vi "To and From CSV.vi"() -> (0 "error out":errorcluster, 1 "Pass":bool, 2 "Lines Equal":bool, 3 "Class Equal":bool)   [LabVIEW 2017, in "J1939 tests.lvlib"]
uses:
  J1939 tests.lvlib
  <vilib>/NI/DCAF/Engines/Standard Engine/Execution Engine/Configuration/Standard Engine Configuration.lvclass
  C:/Program Files (x86)/National Instruments/LabVIEW 2017/vi.lib/NI/Module Execution Interface/Engine Configuration/engine configuration.lvclass
  editor node/J1939 editor node.lvclass
  module/configuration/J1939 configuration.lvclass
  C:/Program Files (x86)/National Instruments/LabVIEW 2017/vi.lib/NI/Configuration Framework/serializable configuration/NISE_CEF_serializable configuration.lvclass
  module/configuration/J1939 configuration.lvclass/J1939 configuration.ctl
  <vilib>/NI/Configuration Framework/serializable configuration/NISE_CEF_serializable configuration.lvclass/NISE_CEF_serializable configuration.ctl
  <vilib>/NI/Tag Bus/tag/tag descriptor.lvclass/tag descriptor.ctl
  <vilib>/NI/Tag Bus Module Framework/channel/TBM channel.lvclass
  C:/Program Files (x86)/National Instruments/LabVIEW 2017/vi.lib/NI/Tag Bus/tag/tag descriptor.lvclass
  <vilib>/Utility/LVClass/Get LV Class Name.vi
  <vilib>/NI/Configuration Framework/error generator/NISE_error generator.vi
  <vilib>/NI/Module Execution Interface/Engine Configuration/engine configuration.lvclass
  <vilib>/NI/Configuration Framework/serializable configuration/NISE_CEF_serializable configuration.lvclass
  <vilib>/NI/Tag Bus/tag/tag descriptor.lvclass
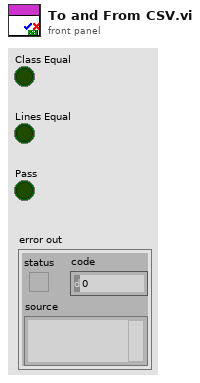
[diagram p1: front panel]
types:
  T1 = typedef "J1939 configuration.lvclass/Line.ctl" = cluster{"channel":refnum<class "TBM channel.lvclass">, "XNET Signal":refnum<k21>}
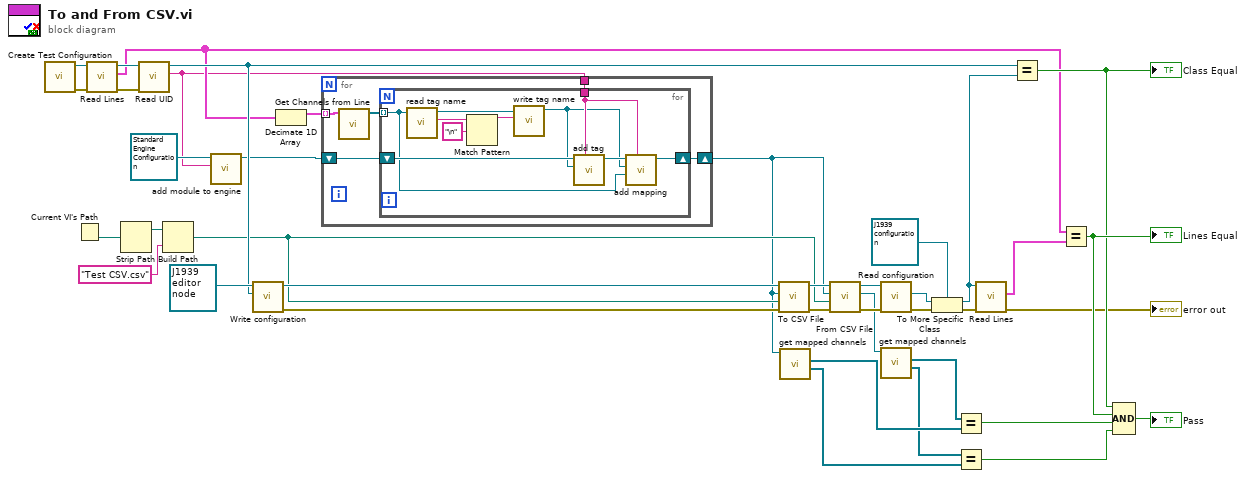
[diagram p0: block diagram]
diagram:
  n1 = call "Create Test Configuration.vi"() -> ("error out"=w14:errorcluster, "Module Configuration"=w39:refnum<class "J1939 configuration.lvclass">)  [unwired: 5 in, 5 out]
  n2 = Current VI's Path() -> (path=w21:path)
  n3 = call "Read Lines.vi"("error in (no error)"=w14, "J1939 configuration in"=w39) -> ("error out"=w13:errorcluster, "Lines"=w5:T1[], "J1939 configuration out"=w34:refnum<class "J1939 configuration.lvclass">)  [unwired: 7 in]
  n4 = Strip Path(path=w21) -> (stripped path=w20:path)  [unwired: 1 out]
  n5 = call <vilib>:"Read UID.vi"("error in"=w13, "configuration in"=w34) -> ("instance id"=w1:string, "configuration out"=w30:refnum<class "J1939 configuration.lvclass">)  [unwired: 7 in, 1 out]
  n6 = Build Path(base path=w20, name or relative path="Test CSV.csv") -> (appended path=w18:path)
  n7 = call-dynamic "add module to engine.vi"("module ID"=w1, "Standard Engine Configuration in"=refnum<class "Standard Engine Configuration.lvclass"> refnum) -> ("Standard Engine Configuration out"=w3:refnum<class "Standard Engine Configuration.lvclass">)  [unwired: 8 in, 1 out]
  n8 = call-dynamic "Write configuration.vi"("configuration"=w30, "J1939 editor node in"=refnum<class "J1939 editor node.lvclass"> refnum ("J1939 editor node")) -> ("error out"=w16:errorcluster, "J1939 editor node out"=w32:refnum<class "J1939 editor node.lvclass">)  [unwired: 8 in]
  n9 = Decimate 1D Array(w5) -> (w4:T1[])  [unwired: 1 out]
  n10 = for {
    tunnel: w4 -> [w44] mode=indexing
    shift-right: [w42] -> w2
    shift-left: w3 -> [w43]
    tunnel: w1 -> [w40]
    n11 = call "Get Channels from Line.vi"("Line"=w44) -> ("Channels"=w41:refnum<class "TBM channel.lvclass">[])  [unwired: 10 in]
    n12 = for {
      tunnel: w41 -> [w48] mode=indexing
      shift-right: [w51] -> w42
      shift-left: w43 -> [w54]
      tunnel: w40 -> [w50]
      n13 = call <vilib>:"read tag name.vi"("system tag in"=w48) -> ("name"=w46:string, "system tag out"=w53:refnum<class "TBM channel.lvclass">)  [unwired: 8 in, 1 out]
      n14 = Match Pattern(string=w46, regular expression="\n" ("search string/char (-)")) -> (before substring=w45:string)  [unwired: 1 in, 3 out]
      n15 = call <vilib>:"write tag name.vi"("name"=w45, "system tag in"=w53) -> ("system tag out"=w49:refnum<class "TBM channel.lvclass">)  [unwired: 8 in, 1 out]
      n16 = call-dynamic "add tag.vi"("owner ID"=w50, "tag descriptor"=w49, "engine configuration in"=w54) -> ("engine configuration out"=w52:refnum<class "Standard Engine Configuration.lvclass">)  [unwired: 7 in, 1 out]
      n17 = call-dynamic "add mapping.vi"("owner ID"=w50, "channel"=w48, "tag descriptor"=w49, "engine configuration"=w52) -> ("engine configuration out"=w51:refnum<class "Standard Engine Configuration.lvclass">)  [unwired: 6 in, 1 out]
    }
  }
  n18 = call-dynamic "To CSV File.vi"("error in (no error)"=w16, "Path"=w18, "engine configuration"=w2, "J1939 editor node in"=w32) -> ("error out"=w37:errorcluster, "J1939 editor node out"=w38:refnum<class "J1939 editor node.lvclass">)  [unwired: 6 in]
  n19 = call-dynamic "get mapped channels.vi"("engine configuration in"=w2) -> ("write channels"=w9:refnum<class "TBM channel.lvclass">[], "read channels"=w11:refnum<class "TBM channel.lvclass">[])  [unwired: 6 in, 3 out]
  n20 = call-dynamic "From CSV File.vi"("error in (no error)"=w37, "Path"=w18, "engine in"=w2, "J1939 editor node in"=w38) -> ("error out"=w17:errorcluster, "engine out"=w12:refnum<class "engine configuration.lvclass">, "J1939 editor node out"=w31:refnum<class "J1939 editor node.lvclass">)  [unwired: 4 in, 1 out]
  n21 = call-dynamic "Read configuration.vi"("error in"=w17, "J1939 editor node in"=w31) -> ("error out"=w25:errorcluster, "configuration"=w28:refnum<class "NISE_CEF_serializable configuration.lvclass">)  [unwired: 7 in, 1 out]
  n22 = call-dynamic "get mapped channels.vi"("engine configuration in"=w12) -> ("write channels"=w8:refnum<class "TBM channel.lvclass">[], "read channels"=w10:refnum<class "TBM channel.lvclass">[])  [unwired: 6 in, 3 out]
  n23 = To More Specific Class(target class=refnum<class "J1939 configuration.lvclass"> refnum ("J1939 configuration out"), reference=w28, error in=w25) -> (specific class reference=w27:refnum<class "J1939 configuration.lvclass">, error out=w26:errorcluster)
  n24 = Equal?(x=w10, y=w11) -> (x = y?=w7:bool)
  n25 = Equal?(x=w8, y=w9) -> (x = y?=w6:bool)
  n26 = call "Read Lines.vi"("error in (no error)"=w26, "J1939 configuration in"=w27) -> ("error out"=→"error out":errorcluster, "Lines"=w35:T1[])  [unwired: 7 in, 1 out]
  n27 = Equal?(x=w30, y=w27) -> (x = y?=w22:bool)
  "Class Equal" <- w22
  n28 = Equal?(x=w5, y=w35) -> (x = y?=w24:bool)
  "Lines Equal" <- w24
  n29 = Compound Arithmetic op=AND(w22, w24, w7, w6) -> (→"Pass":bool)
